vi "Sensor_Values.vi"() -> ()   [LabVIEW 2020]
panel:
  out "Magazine_Loaded":bool
  in  "Outer_Arm_Pivot_Position(ticks)":i32
  in  "Inner_Arm_Pivot_Position(ticks)":i32
  in  "Outer_Arm_Elevator_Position (ticks)":i32
  in  "Safe_Module_Latch_Angle(deg)":dbl
  in  "Pose_Loop_Time(ms)":u32
  in  "Robot_Ground_Speed(ft/s)":dbl
  in  "Robot_Y_Position(in)":dbl
  in  "Robot_X_Position(in)":dbl
  in  "Turret_Absolute_Zero":i32
  in  "Flywheel_Velocity(RPM)":dbl
  in  "Camera_Goal_Area":dbl
  in  "Camera_Goal_X":dbl
  out "Zero_Turret_Spin":bool
  in  "Flywheel_Right_Velocity":dbl
  in  "Flywheel_Left_Velocity":dbl
  in  "Turret_Relative_Position(Native Units)":i32
  in  "Camera_X_Offset":dbl
  in  "Turret_Absolute_Position(Degrees)":dbl
  in  "Camera_Area":dbl
  in  "Drive_IMU (deg)":dbl
  in  "Back_Right_Wheel_Angle (deg)":dbl
  in  "Back_Left_Wheel_Angle (deg)":dbl
  in  "Front_Left_Wheel_Angle (deg)":dbl
  in  "Front_Right_Wheel_Angle (deg)":dbl
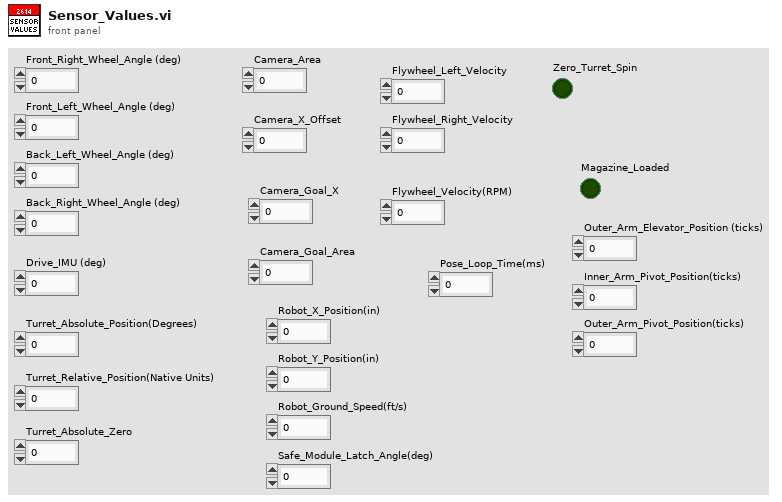
[diagram p1: front panel]
diagram:
